vi "Check Used Types.vi"(8 "error in (no error)":errorcluster, 10 "Message":T1, 11 "LV-Protoc in":refnum<class "LV-Protoc.lvclass">) -> (0 "error out":errorcluster, 3 "LV-Protoc out":refnum<class "LV-Protoc.lvclass">)   [LabVIEW 2020, in "LV-Protoc.lvlib" / "LV-Protoc.lvclass"]
uses:
  LV-Protoc.lvclass
  LV-Proto/Message.ctl
  LV-Proto/Field.ctl
  LV-Proto/Type.ctl
  LV-Proto/Proto Type.ctl
  LV-Protoc.lvclass/LV-Protoc.ctl
  LV-Proto/LV-Proto.lvlib
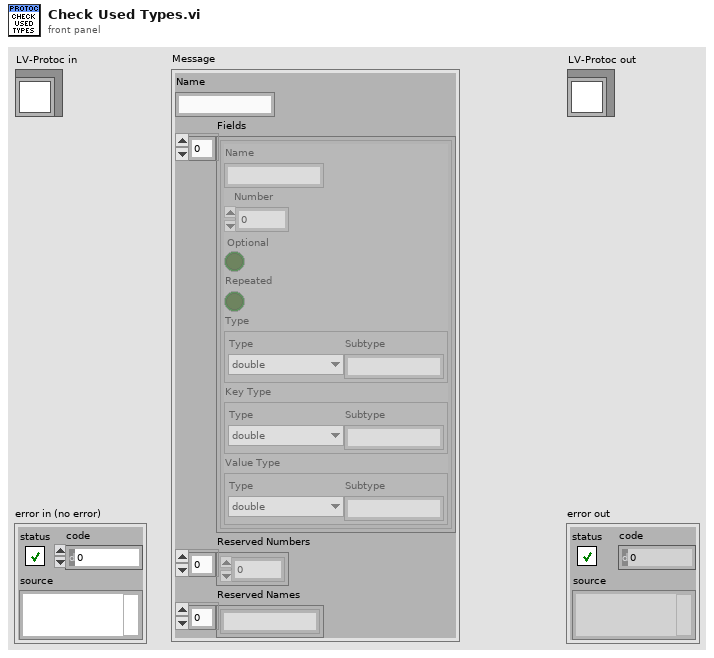
[diagram p1: front panel]
types:
  T1 = typedef "LV-Proto.lvlib/Message.ctl" = cluster{"Name":string, "Fields":T2[], "Reserved Numbers":u32[], "Reserved Names":string[]}
  T2 = typedef "LV-Proto.lvlib/Field.ctl" = cluster{"Name":string, "Number":u32, "Optional":bool, "Repeated":bool, "Type":T3, "Key Type":T3, "Value Type":T3}
  T3 = typedef "LV-Proto.lvlib/Type.ctl" = cluster{"Type":T4, "Subtype":string}
  T4 = typedef "LV-Proto.lvlib/Proto Type.ctl" = enum16{"UNKNOWN", "double", "float", "int32", "int64", "uint32", "uint64", "sint32", "sint64", "fixed32", "fixed64", "sfixed32", "sfixed64", "bool", "string", "bytes", "enum", "map", "message"}
  T5 = typedef "LV-Protoc.lvlib/Enumeration Paths.ctl" = cluster{"Name":string, "Library":path, "Typedef":path, "Encode":path, "Encode packed":path, "Decode":path, "Decode packed":path, "Enum Value":path, "Enum from Value":path}
  T6 = typedef "LV-Protoc.lvlib/Message Paths.ctl" = cluster{"Name":string, "Library":path, "Data Typedef":path, "MessageName VI":path, "Flatten VI":path, "Unflatten VI":path, "Flatten repeated VI":path, "Decode VI":path}
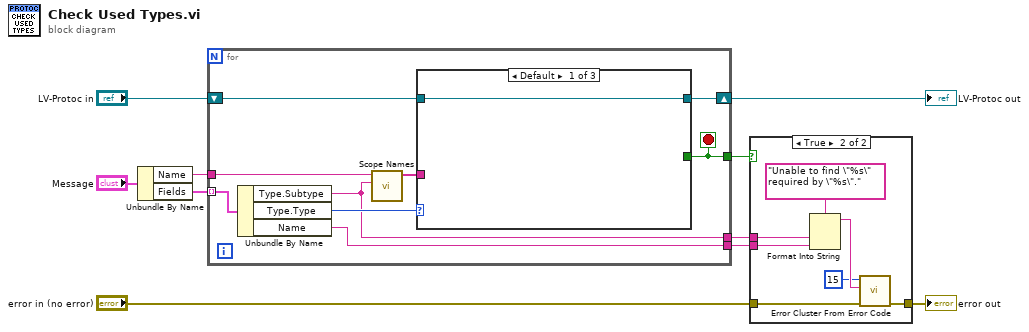
[diagram p0: block diagram]
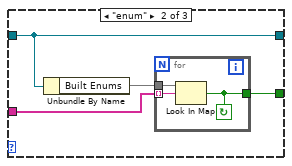
[diagram p3: hidden frame]
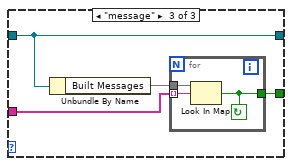
[diagram p4: hidden frame]
diagram:
  n1 = Unbundle By Name("Message") -> ("Name"=w6:string, "Fields"=w7:T2[])
  n2 = for {
    shift-right: [w14] -> w8
    shift-left: "LV-Protoc in" -> [w17]
    tunnel: w7 -> [w19] mode=indexing
    tunnel: w6 -> [w16]
    tunnel: [w13] -> w5
    tunnel: [w12] -> w4
    tunnel: [w11] -> w3
    stop <- w13 stop-if-true
    n3 = Unbundle By Name(w19) -> ("Type.Subtype"=w11:string, "Type.Type"=w18:T4, "Name"=w12:string)
    n4 = call "Scope Names.vi"("Type Name"=w11, "Container Name"=w16) -> ("Scope Names"=w15:string[])  [unwired: 9 in]
    n5 = case shown="Default" w18 {
      tunnel: w17 -> [w20 w22 w29]
      tunnel: w15 -> [_ w23 w30]
      tunnel: [w20 w22 w29] -> w14
      tunnel: [_ w21 w28] -> w13
      frame Default {
      }
      frame "enum" {
        n6 = Unbundle By Name(w22) -> ("Built Enums"=w24:map{string, T5})
        n7 = for {
          tunnel: w24 -> [w27]
          tunnel: w23 -> [w26] mode=indexing
          tunnel: [w25] -> w21
          stop <- w25 continue-if-true
          n8 = Look In Map(map=w27, key=w26) -> (key not found?=w25:bool)  [unwired: 1 in, 1 out]
        }
      }
      frame "message" {
        n9 = Unbundle By Name(w29) -> ("Built Messages"=w31:map{string, T6})
        n10 = for {
          tunnel: w31 -> [w34]
          tunnel: w30 -> [w33] mode=indexing
          tunnel: [w32] -> w28
          stop <- w32 continue-if-true
          n11 = Look In Map(map=w34, key=w33) -> (key not found?=w32:bool)  [unwired: 1 in, 1 out]
        }
      }
    }
  }
  "LV-Protoc out" <- w8
  n12 = case shown="True" w5 {
    tunnel: w4 -> [_ w40]
    tunnel: w3 -> [_ w41]
    tunnel: "error in (no error)" -> [w35 w37]
    tunnel: [w35 w36] -> w1
    frame False {
    }
    frame True {
      n13 = Format Into String(format string="Unable to find \"%s\" required by \"%s\".", w41, w40) -> (resulting string=w39:string)  [unwired: 2 in, 1 out]
      n14 = call <vilib>:"Error Cluster From Error Code.vi"("error in (no error)"=w37, "error message (\"\")"=w39, "error code (0)"=15) -> ("error out"=w36:errorcluster)  [unwired: 6 in]
    }
  }
  "error out" <- w1
